vi "CreateWaveformArray.vi"(4 "error in (no error)":errorcluster, 6 "bufferSize":dbl) -> (0 "error out":errorcluster, 2 "initialized array":waveform(dbl)[](array[waveform]))   [LabVIEW 2016]
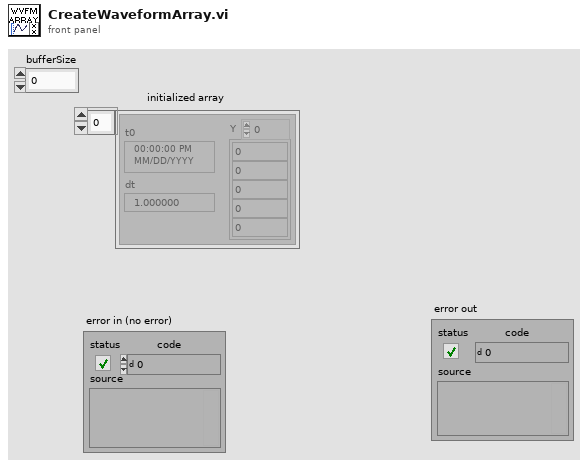
[diagram p1: front panel]
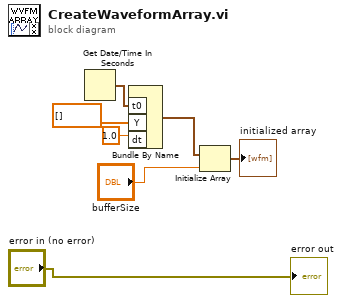
[diagram p0: block diagram]
diagram:
  n1 = Get Date/Time In Seconds() -> (seconds since 1Jan1904=w4:timestamp)
  n2 = Bundle By Name("t0"=w4, "Y"=dbl[] [], "dt"=1.0) -> (w7:waveform(dbl))  [unwired: 1 in]
  n3 = Initialize Array(w7, "bufferSize") -> (→"initialized array":waveform(dbl)[])
  "error out" <- "error in (no error)"
